vi "Input Zero.vi"(8 "error in (no error)":errorcluster, 9 "Timeout Value (350000)":u32=350000, 10 "Input Zero (0: Single Range)":u16(ring) items=["Single Range", "Multiple Range"], 11 "VISA resource name":refnum<visa-resource-name>) -> (0 "error out":errorcluster, 2 "Input Zero Pass?":bool, 3 "VISA resource name out":refnum<visa-resource-name>)   [LabVIEW 2012, in "Fluke 8508.lvlib"]
doc: "This VI determines and corrects for the input zero and stores the result in volatile memory. An Input Zero is stored only for the input channel selected. Each input has its own set of Input Zero stores, for all of the applicable range/function combinations. For the OHMS function, an independent Input Zero should be executed for the two/four wire connection and for the low/normal current selection. The PRT function utilizes input zero’s obtained in the relevant OHMS/TRUE OHMS ranges.\n\nNOTES:\n(1) The Input Zero operation can take several seconds to complete.\n(2) An error will be generated if calibration is enabled, the PRT function is selected or a scan operation is selected."
uses:
  Fluke 8508.lvlib
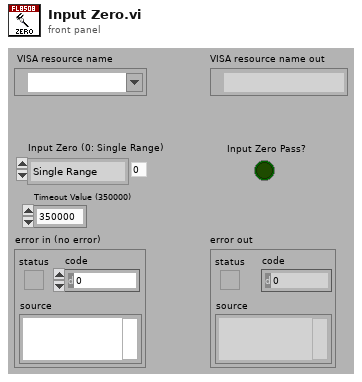
[diagram p1: front panel]
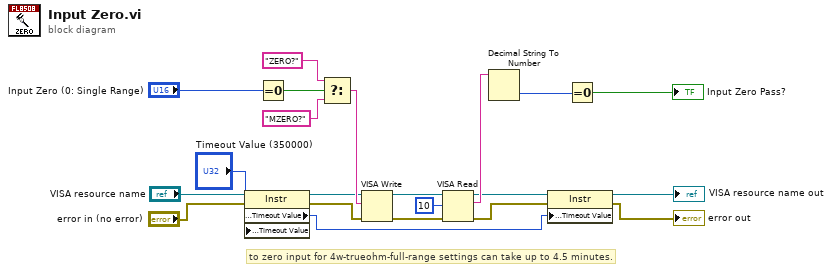
[diagram p0: block diagram]
diagram:
  # "to zero input for 4w-trueohm-full-range settings can take up to 4.5 minutes."
  n1 = property class="Instr"(reference="VISA resource name", error in="error in (no error)", "General Settings:Timeout Value"="Timeout Value (350000)") -> (reference out=w8:refnum<visa-resource-name>, error out=w7:errorcluster, "General Settings:Timeout Value"=w2:u32)
  n2 = Equal To 0?(x="Input Zero (0: Single Range)") -> (x = 0?=w20:bool)
  n3 = Select(t="ZERO?", s=w20, f="MZERO?") -> (s? t:f=w17:string)
  n4 = VISA Write(VISA resource name=w8, write buffer=w17, error in (no error)=w7) -> (VISA resource name out=w16:refnum<visa-resource-name>, error out=w15:errorcluster)  [unwired: 1 out]
  n5 = VISA Read(VISA resource name=w16, byte count=u32 10, error in (no error)=w15) -> (VISA resource name out=w6:refnum<visa-resource-name>, read buffer=w11:string, error out=w4:errorcluster)  [unwired: 1 out]
  n6 = Decimal String To Number(string=w11) -> (number=w12:i32)  [unwired: 2 in, 1 out]
  n7 = property class="Instr"(reference=w6, error in=w4, "General Settings:Timeout Value"=w2) -> (reference out=→"VISA resource name out":refnum<visa-resource-name>, error out=→"error out":errorcluster)
  n8 = Equal To 0?(x=w12) -> (x = 0?=→"Input Zero Pass?":bool)
